vi "Format Alarm Data.vi"(5 "Area color settings":T3(array[cluster]), 7 "Alarm Display Format":T2(array[ring])=[enum."alarm URL", enum."set time", enum."set point", enum."value", enum."alarm description"], 8 "Error In":errorcluster, 10 "alarm instances":T1(array[cluster]), 11 "Multicolumn Listbox":refnum<vi>) -> (0 "Error Out":errorcluster, 1 "Alarm Summary Data":string[][](array[string]), 2 "Alarm Summary Headers":string[](array[string]), 3 "dup Multicolumn Listbox":refnum<vi>)   [LabVIEW 2013]
doc: "This VI formats alarm data and inserts it into a multicolumn list box."
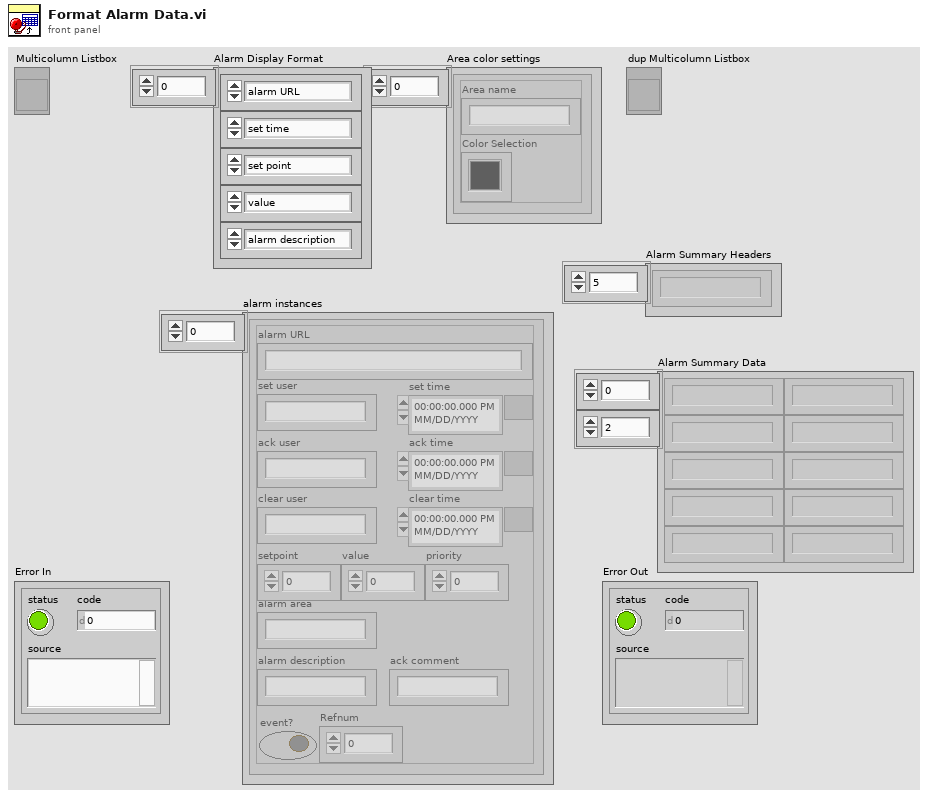
[diagram p1: front panel]
types:
  T1 = cluster{"alarm URL":string, "set time":timestamp, "set user":string, "ack time":timestamp, "ack user":string, "clear time":timestamp, "clear user":string, "setpoint":dbl, "value":dbl, "priority":u32, "alarm area":string, "alarm description":string, "ack comment":string, "event?":bool, "Refnum":u64}[]
  T2 = enum16{"alarm URL", "event?", "set time", "ack time", "clear time", "set user", "ack user", "clear user", "set point", "value", "priority", "alarm area", "alarm description", "ack comment"}[]
  T3 = cluster{"Area name":string, "Color Selection":u32}[]
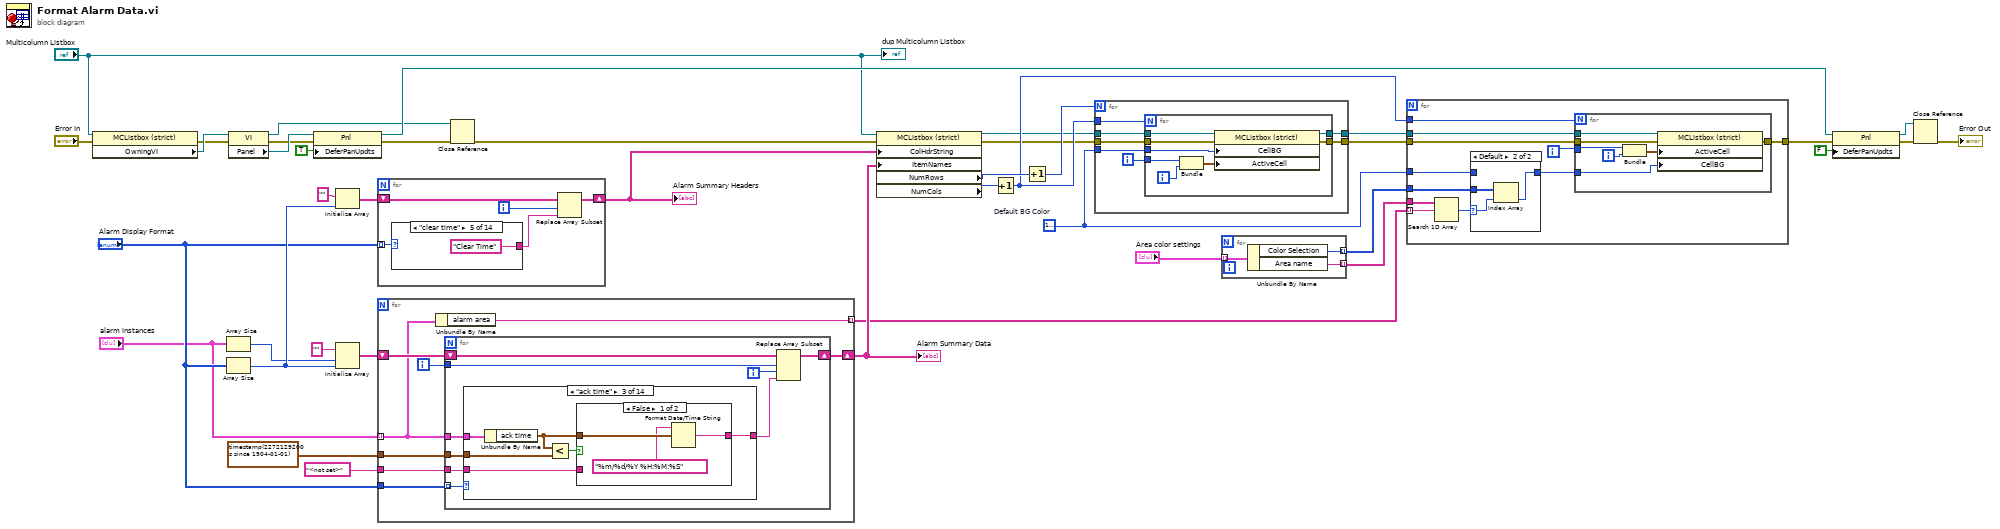
[diagram p0: block diagram]
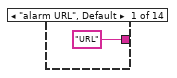
[diagram p3: hidden frame]
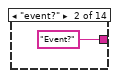
[diagram p4: hidden frame]
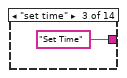
[diagram p5: hidden frame]
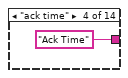
[diagram p6: hidden frame]
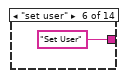
[diagram p7: hidden frame]
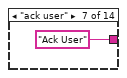
[diagram p8: hidden frame]
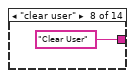
[diagram p9: hidden frame]
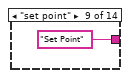
[diagram p10: hidden frame]
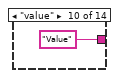
[diagram p11: hidden frame]
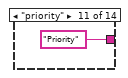
[diagram p12: hidden frame]
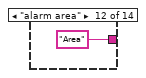
[diagram p13: hidden frame]
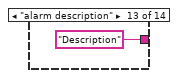
[diagram p14: hidden frame]
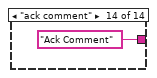
[diagram p15: hidden frame]
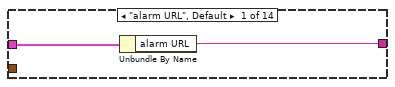
[diagram p16: hidden frame]
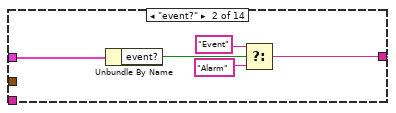
[diagram p17: hidden frame]
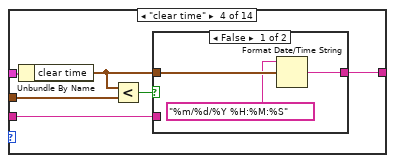
[diagram p19: hidden frame]
diagram:
  w4 = u32 16777226  # Default BG Color
  n1 = property class="MCListbox (strict)"(reference="Multicolumn Listbox", error in="Error In") -> (error out=w18:errorcluster, "OwningVI"=w19:refnum<vi>)  [unwired: 1 out]
  n2 = Array Size(array="alarm instances") -> (size(s)=w33:i32)
  n3 = Array Size(array="Alarm Display Format") -> (size(s)=w38:i32)
  n4 = property class="VI"(reference=w19, error in=w18) -> (reference out=w11:refnum<vi>, error out=w16:errorcluster, "Panel"=w17:refnum<vi>)
  n5 = property class="Pnl"(reference=w17, error in=w16, "DeferPanUpdts"=TRUE ("Defer Panel Updates")) -> (reference out=w12:refnum<vi>, error out=w10:errorcluster)
  n6 = Initialize Array("" ("element"), w38) -> (w39:string[])
  n7 = Initialize Array("" ("alarm URL"), w33, w38) -> (w35:string[][])
  n8 = for {
    tunnel: "alarm instances" -> [w43] mode=indexing
    tunnel: "Alarm Display Format" -> [w49]
    shift-right: [w47] -> w40
    shift-left: w35 -> [w48]
    tunnel: timestamp(2272129200 s since 1904-01-01) ("ack time") -> [w45]
    tunnel: "<not set>" ("date/time string") -> [w44]
    tunnel: [w42] -> w29 mode=indexing
    i -> [w46]
    n9 = Unbundle By Name(w43) -> ("alarm area"=w42:string)
    n10 = for {
      tunnel: w49 -> [w58] mode=indexing
      tunnel: w43 -> [w50]
      tunnel: w46 -> [w55]
      shift-right: [w56] -> w47
      shift-left: w48 -> [w57]
      tunnel: w45 -> [w52]
      tunnel: w44 -> [w51]
      i -> [w54]
      n11 = case shown="\"ack time\"" w58 {
        tunnel: w50 -> [w60 w65 w71 w81 w91 w97 w99 w101 w104 w107 w110 w112 w114 w116]
        tunnel: [w59 w61 w70 w80 w90 w96 w98 w100 w102 w105 w108 w111 w113 w115] -> w53
        tunnel: w52 -> [_ _ w68 w78 w88 _ _ _ _ _ _ _ _ _]
        tunnel: w51 -> [_ _ w66 w76 w86 _ _ _ _ _ _ _ _ _]
        frame "alarm URL", Default {
          n12 = Unbundle By Name(w60) -> ("alarm URL"=w59:string)
        }
        frame "event?" {
          n13 = Unbundle By Name(w65) -> ("event?"=w64:bool)
          n14 = Select(t="Event" ("alarm URL"), s=w64, f="Alarm") -> (s? t:f=w61:string)
        }
        frame "ack time" {
          n15 = Unbundle By Name(w71) -> ("ack time"=w67:timestamp)
          n16 = Less?(x=w67, y=w68) -> (x < y?=w69:bool)
          n17 = case shown="False" w69 {
            tunnel: w67 -> [w74 _]
            tunnel: [w72 w75] -> w70
            tunnel: w66 -> [_ w75]
            frame False {
              n18 = Format Date/Time String(time format string (%c)="%m/%d/%Y %H:%M:%S", seconds (now)=w74) -> (date/time string=w72:string)  [unwired: 1 in]
            }
            frame True {
            }
          }
        }
        frame "clear time" {
          n19 = Unbundle By Name(w81) -> ("clear time"=w77:timestamp)
          n20 = Less?(x=w77, y=w78) -> (x < y?=w79:bool)
          n21 = case shown="False" w79 {
            tunnel: w77 -> [w84 _]
            tunnel: [w82 w85] -> w80
            tunnel: w76 -> [_ w85]
            frame False {
              n22 = Format Date/Time String(time format string (%c)="%m/%d/%Y %H:%M:%S", seconds (now)=w84) -> (date/time string=w82:string)  [unwired: 1 in]
            }
            frame True {
            }
          }
        }
        frame "set time" {
          n23 = Unbundle By Name(w91) -> ("set time"=w87:timestamp)
          n24 = Less?(x=w87, y=w88) -> (x < y?=w89:bool)
          n25 = case shown="False" w89 {
            tunnel: w87 -> [w94 _]
            tunnel: [w92 w95] -> w90
            tunnel: w86 -> [_ w95]
            frame False {
              n26 = Format Date/Time String(time format string (%c)="%m/%d/%Y %H:%M:%S", seconds (now)=w94) -> (date/time string=w92:string)  [unwired: 1 in]
            }
            frame True {
            }
          }
        }
        frame "set user" {
          n27 = Unbundle By Name(w97) -> ("set user"=w96:string)
        }
        frame "ack user" {
          n28 = Unbundle By Name(w99) -> ("ack user"=w98:string)
        }
        frame "clear user" {
          n29 = Unbundle By Name(w101) -> ("ack user"=w100:string)
        }
        frame "set point" {
          n30 = Unbundle By Name(w104) -> ("setpoint"=w103:dbl)
          n31 = Number To Fractional String(number=w103) -> (F-format string=w102:string)  [unwired: 3 in]
        }
        frame "value" {
          n32 = Unbundle By Name(w107) -> ("value"=w106:dbl)
          n33 = Number To Fractional String(number=w106) -> (F-format string=w105:string)  [unwired: 3 in]
        }
        frame "priority" {
          n34 = Unbundle By Name(w110) -> ("priority"=w109:u32)
          n35 = Number To Decimal String(number=w109) -> (decimal integer string=w108:string)  [unwired: 1 in]
        }
        frame "alarm area" {
          n36 = Unbundle By Name(w112) -> ("alarm area"=w111:string)
        }
        frame "alarm description" {
          n37 = Unbundle By Name(w114) -> ("alarm description"=w113:string)
        }
        frame "ack comment" {
          n38 = Unbundle By Name(w116) -> ("ack comment"=w115:string)
        }
      }
      n39 = Replace Array Subset(array=w57, new element=w53, index (row)=w55, index (col)=w54) -> (w56:string[][])
    }
  }
  "Alarm Summary Data" <- w40
  n40 = for {
    tunnel: "Alarm Display Format" -> [w121] mode=indexing
    shift-right: [w119] -> w41
    shift-left: w39 -> [w120]
    i -> [w118]
    n41 = case shown="\"clear time\"" w121 {
      tunnel: ["URL" ("element") "Event?" ("element") "Set Time" ("element") "Ack Time" ("element") "Clear Time" ("element") "Set User" ("element") "Ack User" ("element") "Clear User" ("element") "Set Point" ("element") "Value" ("element") "Priority" ("element") "Area" ("element") "Description" ("element") "Ack Comment" ("element")] -> w117
      frame "alarm URL", Default {
      }
      frame "event?" {
      }
      frame "set time" {
      }
      frame "ack time" {
      }
      frame "clear time" {
      }
      frame "set user" {
      }
      frame "ack user" {
      }
      frame "clear user" {
      }
      frame "set point" {
      }
      frame "value" {
      }
      frame "priority" {
      }
      frame "alarm area" {
      }
      frame "alarm description" {
      }
      frame "ack comment" {
      }
    }
    n42 = Replace Array Subset(array=w120, new element=w117, index=w118) -> (w119:string[])
  }
  "Alarm Summary Headers" <- w41
  n43 = Close Reference(reference=w11, error in (no error)=w10) -> (error out=w9:errorcluster)
  n44 = property class="MCListbox (strict)"(reference="Multicolumn Listbox", error in=w9, "ColHdrString"=w41, "ItemNames"=w40) -> (reference out=w20:refnum<vi>, error out=w6:errorcluster, "NumRows"=w24:u32, "NumCols"=w25:u32)
  n45 = Increment(x=w25) -> (x+1=w22:u32)
  n46 = Increment(x=w24) -> (x+1=w23:u32)
  n47 = for {
    N: w23 -> [_]
    tunnel: [w141] -> w21
    tunnel: w22 -> [w140]
    tunnel: w20 -> [w139]
    tunnel: w4 -> [w138]
    tunnel: w6 -> [w137]
    tunnel: [w136] -> w5
    i -> [w142]
    n48 = for {
      N: w140 -> [_]
      tunnel: w142 -> [w150]
      tunnel: [w149] -> w141
      tunnel: w139 -> [w147]
      tunnel: w138 -> [w146]
      tunnel: w137 -> [w145]
      tunnel: [w144] -> w136
      i -> [w148]
      n49 = Bundle(w150, w148) -> (w143:cluster{i32, i32})  [unwired: 1 in]
      n50 = property class="MCListbox (strict)"(reference=w147, error in=w145, "CellBG"=w146, "ActiveCell"=w143) -> (reference out=w144:refnum<vi>, error out=w149:errorcluster)
    }
  }
  n51 = for {
    tunnel: "Area color settings" -> [w153] mode=indexing
    tunnel: [w152] -> w27 mode=indexing
    tunnel: [w151] -> w26 mode=indexing
    n52 = Unbundle By Name(w153) -> ("Color Selection"=w151:u32, "Area name"=w152:string)
  }
  n53 = for {
    tunnel: w5 -> [w164]
    tunnel: w29 -> [w160] mode=indexing
    tunnel: [w163] -> w13
    tunnel: w22 -> [w162]
    tunnel: w27 -> [w161]
    tunnel: w26 -> [w159]
    tunnel: w21 -> [w155]
    tunnel: w4 -> [w156]
    i -> [w154]
    n54 = Search 1D Array(1D array=w161, element=w160) -> (index of element=w157:i32)  [unwired: 1 in]
    n55 = case shown="Default" w157 {
      selector: w157 -> [_ w166]
      tunnel: w159 -> [_ w168]
      tunnel: [w165 w167] -> w158
      tunnel: w156 -> [w165 _]
      frame ..-1 {
      }
      frame Default {
        n56 = Index Array(array=w168, index=w166) -> (element=w167:u32)
      }
    }
    n57 = for {
      N: w162 -> [_]
      tunnel: w164 -> [w175]
      tunnel: w154 -> [w174]
      tunnel: [w173] -> w163
      tunnel: w158 -> [w170]
      tunnel: w155 -> [w169]
      i -> [w172]
      n58 = Bundle(w174, w172) -> (w171:cluster{i32, i32})  [unwired: 1 in]
      n59 = property class="MCListbox (strict)"(reference=w175, error in=w169, "ActiveCell"=w171, "CellBG"=w170) -> (error out=w173:errorcluster)  [unwired: 1 out]
    }
  }
  n60 = property class="Pnl"(reference=w12, error in=w13, "DeferPanUpdts"=FALSE ("Defer Panel Updates")) -> (reference out=w7:refnum<vi>, error out=w8:errorcluster)
  n61 = Close Reference(reference=w7, error in (no error)=w8) -> (error out=→"Error Out":errorcluster)
  "dup Multicolumn Listbox" <- "Multicolumn Listbox"
